vi "I2C LCD Full.vi"() -> ()   [LabVIEW 2023, in "CTI-Visa-Scratchpad.lvlib"]
uses:
  CTI-Visa-Scratchpad.lvlib
  CTI-Visa-DeviceLib/LCD-I2C/Position.ctl
  CTI-Visa-DeviceLib/LCD-I2C/LCD Size.ctl
  CTI-Visa/I2C Options.ctl
  CTI-Visa-DeviceLib/LCD-I2C/Custom Char.ctl
  CTI-Visa/CTI-Visa.lvlib
  CTI-Visa-DeviceLib/LCD-I2C/LCD-I2C.lvclass
panel:
  in  "Custom Chars":T2
  in  "Backlight":bool=TRUE
  in  "Create":bool
  in  "Address":u8=39 format="%.0x"
  in  "I2C Options":T3={"Bus"=0, "Baud"=400000, "SCL GPIO"=16, "SDA GPIO"=17}
  in  "LCD Size":T4={"Rows"=2, "Cols"=16}
  in  "stop":bool
  out "error out":errorcluster
  in  "Scroll Right":bool
  in  "Scroll Left":bool
  in  "Home":bool
  in  "Clear":bool
  in  "Write Text":bool
  in  "Text":string="Hello LabVIEW!"
  in  "Port":refnum<visa-resource-name>="COM4"
  in  "Goto":bool
  in  "Position":T5
  in  "Display":bool=TRUE
  in  "Blink":bool
  in  "Cursor":bool=TRUE
  # "Use \\00 through \\07 to specify custom chars"
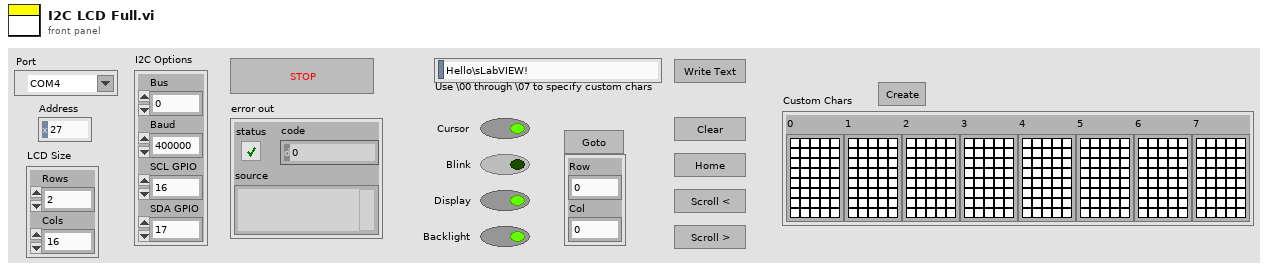
[diagram p1: front panel]
types:
  T1 = typedef "CTI-Visa-DeviceLib.lvlib/LCD-I2C.lvclass/Custom Char.ctl" = bool[][]
  T2 = cluster{"0":T1, "1":T1, "2":T1, "3":T1, "4":T1, "5":T1, "6":T1, "7":T1}
  T3 = typedef "CTI-Visa.lvlib/I2C Options.ctl" = cluster{"Bus":u8, "Baud":u32, "SCL GPIO":i32, "SDA GPIO":i32}
  T4 = typedef "CTI-Visa-DeviceLib.lvlib/LCD-I2C.lvclass/LCD Size.ctl" = cluster{"Rows":u8, "Cols":u8}
  T5 = typedef "CTI-Visa-DeviceLib.lvlib/LCD-I2C.lvclass/Position.ctl" = cluster{"Row":u8, "Col":u8}
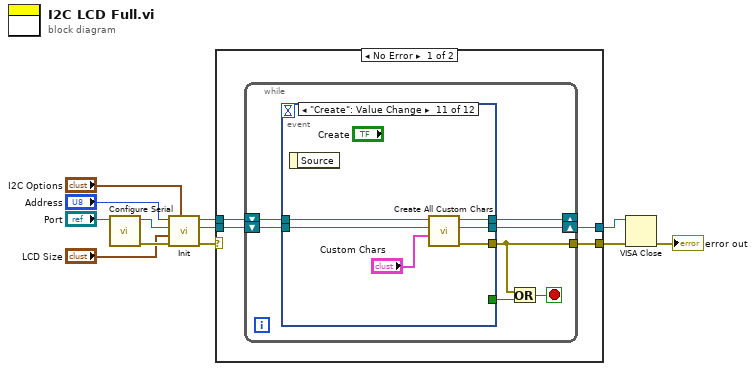
[diagram p0: block diagram]
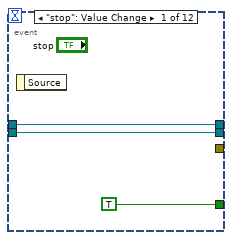
[diagram p2: hidden frame]
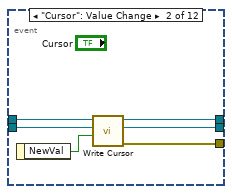
[diagram p3: hidden frame]
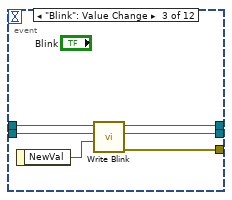
[diagram p4: hidden frame]
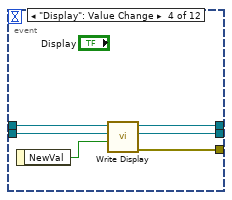
[diagram p5: hidden frame]
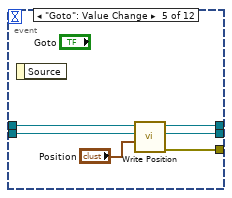
[diagram p6: hidden frame]
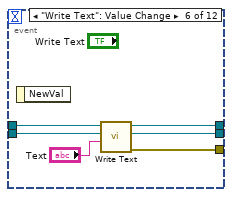
[diagram p7: hidden frame]
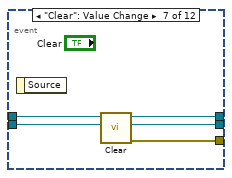
[diagram p8: hidden frame]
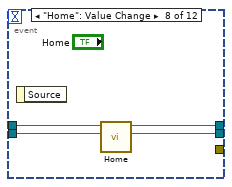
[diagram p9: hidden frame]
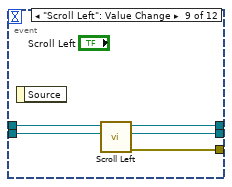
[diagram p10: hidden frame]
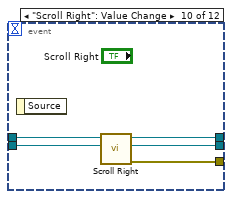
[diagram p11: hidden frame]
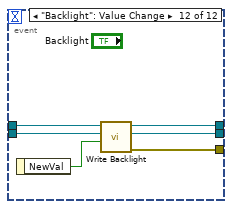
[diagram p12: hidden frame]
diagram:
  n1 = call "Configure Serial.vi"("VISA resource name in"="Port") -> ("error out"=w11:errorcluster, "VISA resource name"=w10:refnum<visa-resource-name>)  [unwired: 9 in]
  n2 = call "Init.vi"("I2C Options"="I2C Options", "error in (no error)"=w11, "LCD Size"="LCD Size", "VISA resource name in"=w10, "Address"="Address") -> ("error out"=w6:errorcluster, "VISA resource name"=w5:refnum<visa-resource-name>, "LCD-I2C out"=w4:refnum<class "LCD-I2C.lvclass">)  [unwired: 4 in]
  n3 = case shown="No Error" w6 {
    selector: w6 -> [_ w88]
    tunnel: w5 -> [w16 w89]
    tunnel: w4 -> [w15 _]
    tunnel: [w14 w89] -> w3
    tunnel: [w13 w88] -> w2
    frame No Error {
      n4 = while {
        shift-right: [w21] -> _
        shift-left: w15 -> [w23]
        shift-right: [w20] -> w14
        shift-left: w16 -> [w22]
        tunnel: [w17] -> w13
        stop <- w18 stop-if-true
        n5 = event shown="[10] \"Create\": Value Change" {
          selector: _ -> [_ _ _ _ _ _ _ _ _ _ _ _]
          dyn-events: _ -> [_ _ _ _ _ _ _ _ _ _ _ _]
          timeout: _ -> [_ _ _ _ _ _ _ _ _ _ _ _]
          tunnel: w23 -> [w26 w31 w38 w44 w50 w56 w61 w65 w70 w74 w78 w84]
          tunnel: w22 -> [w25 w32 w37 w43 w49 w55 w60 w64 w69 w75 w81 w87]
          tunnel: [w26 w30 w36 w42 w46 w53 w59 w62 w67 w72 w80 w85] -> w21
          tunnel: [w25 w29 w35 w41 w45 w52 w58 w63 w68 w73 w79 w86] -> w20
          tunnel: [TRUE _ _ _ _ _ _ _ _ _ _ _] -> w19
          tunnel: [_ w27 w33 w39 w47 w51 w57 _ w66 w71 w77 w82] -> w17
          event "stop": Value Change {
            n6 = event-data() -> ()  [unwired: 1 in, 1 out]
          }
          event "Cursor": Value Change {
            n7 = event-data() -> ("NewVal"=w28:bool)  [unwired: 1 in]
            n8 = call "Write Cursor.vi"("Cursor On"=w28, "VISA resource name in"=w32, "LCD-I2C in"=w31) -> ("error out"=w27:errorcluster, "VISA resource name"=w29:refnum<visa-resource-name>, "LCD-I2C out"=w30:refnum<class "LCD-I2C.lvclass">)  [unwired: 6 in]
          }
          event "Blink": Value Change {
            n9 = event-data() -> ("NewVal"=w34:bool)  [unwired: 1 in]
            n10 = call "Write Blink.vi"("Blink On"=w34, "VISA resource name in"=w37, "LCD-I2C in"=w38) -> ("error out"=w33:errorcluster, "VISA resource name"=w35:refnum<visa-resource-name>, "LCD-I2C out"=w36:refnum<class "LCD-I2C.lvclass">)  [unwired: 6 in]
          }
          event "Display": Value Change {
            n11 = event-data() -> ("NewVal"=w40:bool)  [unwired: 1 in]
            n12 = call "Write Display.vi"("Display On"=w40, "VISA resource name in"=w43, "LCD-I2C in"=w44) -> ("error out"=w39:errorcluster, "VISA resource name"=w41:refnum<visa-resource-name>, "LCD-I2C out"=w42:refnum<class "LCD-I2C.lvclass">)  [unwired: 6 in]
          }
          event "Goto": Value Change {
            n13 = event-data() -> ()  [unwired: 1 in, 1 out]
            n14 = call "Write Position.vi"("Position"="Position", "VISA resource name in"=w49, "LCD-I2C in"=w50) -> ("error out"=w47:errorcluster, "VISA resource name"=w45:refnum<visa-resource-name>, "LCD-I2C out"=w46:refnum<class "LCD-I2C.lvclass">)  [unwired: 6 in]
          }
          event "Write Text": Value Change {
            n15 = event-data() -> ()  [unwired: 1 in, 1 out]
            n16 = call "Write Text.vi"("Text"="Text", "VISA resource name in"=w55, "LCD-I2C in"=w56) -> ("error out"=w51:errorcluster, "VISA resource name"=w52:refnum<visa-resource-name>, "LCD-I2C out"=w53:refnum<class "LCD-I2C.lvclass">)  [unwired: 6 in]
          }
          event "Clear": Value Change {
            n17 = event-data() -> ()  [unwired: 1 in, 1 out]
            n18 = call "Clear.vi"("VISA resource name in"=w60, "LCD-I2C in"=w61) -> ("error out"=w57:errorcluster, "VISA resource name"=w58:refnum<visa-resource-name>, "LCD-I2C out"=w59:refnum<class "LCD-I2C.lvclass">)  [unwired: 7 in]
          }
          event "Home": Value Change {
            n19 = event-data() -> ()  [unwired: 1 in, 1 out]
            n20 = call "Home.vi"("VISA resource name in"=w64, "LCD-I2C in"=w65) -> ("VISA resource name"=w63:refnum<visa-resource-name>, "LCD-I2C out"=w62:refnum<class "LCD-I2C.lvclass">)  [unwired: 7 in, 1 out]
          }
          event "Scroll Left": Value Change {
            n21 = event-data() -> ()  [unwired: 1 in, 1 out]
            n22 = call "Scroll Left.vi"("VISA resource name in"=w69, "LCD-I2C in"=w70) -> ("error out"=w66:errorcluster, "VISA resource name"=w68:refnum<visa-resource-name>, "LCD-I2C out"=w67:refnum<class "LCD-I2C.lvclass">)  [unwired: 7 in]
          }
          event "Scroll Right": Value Change {
            n23 = event-data() -> ()  [unwired: 1 in, 1 out]
            n24 = call "Scroll Right.vi"("VISA resource name in"=w75, "LCD-I2C in"=w74) -> ("error out"=w71:errorcluster, "VISA resource name"=w73:refnum<visa-resource-name>, "LCD-I2C out"=w72:refnum<class "LCD-I2C.lvclass">)  [unwired: 7 in]
          }
          event "Create": Value Change {
            n25 = event-data() -> ()  [unwired: 1 in, 1 out]
            n26 = call "Create All Custom Chars.vi"("All Chars"="Custom Chars", "VISA resource name in"=w81, "LCD-I2C in"=w78) -> ("error out"=w77:errorcluster, "VISA resource name"=w79:refnum<visa-resource-name>, "LCD-I2C out"=w80:refnum<class "LCD-I2C.lvclass">)  [unwired: 6 in]
          }
          event "Backlight": Value Change {
            n27 = event-data() -> ("NewVal"=w83:bool)  [unwired: 1 in]
            n28 = call "Write Backlight.vi"("Backlight On"=w83, "VISA resource name in"=w87, "LCD-I2C in"=w84) -> ("error out"=w82:errorcluster, "VISA resource name"=w86:refnum<visa-resource-name>, "LCD-I2C out"=w85:refnum<class "LCD-I2C.lvclass">)  [unwired: 6 in]
          }
        }
        n29 = Or(x=w17, y=w19) -> (x .or. y?=w18:bool)
      }
    }
    frame Error {
    }
  }
  n30 = VISA Close(VISA resource name=w3, error in (no error)=w2) -> (error out=→"error out":errorcluster)
